vi "PVS Calibration.vi"(8 "Error In":errorcluster, 10 "Config PVS.AVOUT":dbl, 11 "TSM Context":T1) -> (0 "Error Out":errorcluster)   [LabVIEW 2019]
doc: "This VI use for Precision Voltage Source Calibration"
uses:
  <vilib>/NI_TestStand_SemiconductorModule/NI_TestStand_Semiconductor_Module.lvlibp/PinMap/General/SemiconductorModuleContext.ctl
  Common/Instrument Control/DMM/Pin Map/TSM DMM.ctl
  <vilib>/NI_TestStand_SemiconductorModule/NI_TestStand_Semiconductor_Module.lvlibp/PinMap/PinQueryContext/MultiplePinMultipleSessionQueryContext/MultiplePinMultipleSessionQueryContext.lvclass
  Common/Instrument Control/Relay/Pin Map/TSM Relay.ctl
  Common/Instrument Control/DCPower/TSM/TSM SSC DCPower.ctl
  Common/Instrument Control/DCPower/SSC DCPower/SSC DCPower.ctl
  Common/Instrument Control/Shared SubVIs/TSM Pin Abstraction/TSM Pin Information.ctl
  Common/Instrument Control/Shared SubVIs/TSM Pin Abstraction/TSM Pin Type Identifier.ctl
  Common/Instrument Control/Shared SubVIs/TSM Pin Abstraction/TSM Expanded Pin Information.ctl
  Common/Utility/typedefs/set_refdac_param.ctl
  <instrlib>/niDMM/nidmm.llb/niDMM Function.ctl
  <instrlib>/niDMM/nidmm.llb/niDMM Resolution in Digits.ctl
  <vilib>/NI_TestStand_SemiconductorModule/NI_TestStand_Semiconductor_Module.lvlibp/1abvi3w/instr.lib/niSwitch/niswitch.llb/niSwitch Relay Action.ctl
  <vilib>/NI_TestStand_SemiconductorModule/NI_TestStand_Semiconductor_Module.lvlibp
panel:
  out "ADC Voltage Out":dbl[](array[numeric])
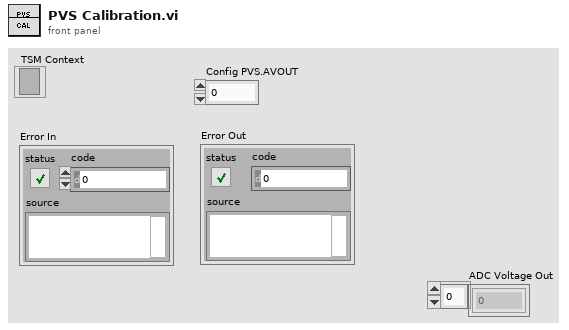
[diagram p1: front panel]
types:
  T1 = typedef "NI_TestStand_Semiconductor_Module.lvlibp/SemiconductorModuleContext.ctl" = refnum<k7>
  T2 = typedef "set_refdac_param.ctl" = cluster{"Read/Write":u16, "VREFP":dbl, "Select Register":enum16{"No Operation", "DAC Register", "Control Register", "Clearcode Register", "Software Control Register"}, "AVOUT ":dbl, "VREFN":dbl}
  T3 = typedef "TSM DMM.ctl" = cluster{"Pin Query Context":refnum<class "MultiplePinMultipleSessionQueryContext.lvclass">, "Sessions":refnum<k15>[]}
  T4 = typedef "TSM Relay.ctl" = cluster{"TSM Context":T1, "Relays":tag[]}
  T5 = typedef "TSM SSC DCPower.ctl" = cluster{"Pin Query Context":refnum<class "MultiplePinMultipleSessionQueryContext.lvclass">, "SSC":T6[], "Site Numbers":i32[], "Pins":T7[], "Pins Expanded":T9[]}
  T6 = typedef "SSC DCPower.ctl" = cluster{"Session":refnum<k15>, "Chan":string, "Channel List":string}
  T7 = typedef "TSM Pin Information.ctl" = cluster{"Pin":tag, "Type":T8, "Count":i32}
  T8 = typedef "TSM Pin Type Identifier.ctl" = enum8{"DUT Pin", "System Pin", "Pin Group", "Not Determined"}
  T9 = typedef "TSM Expanded Pin Information.ctl" = cluster{"Pin":tag, "Type":T8, "Index":i32}
  T10 = cluster{"DMM_Meas":T3, "PVS Cal Relay":T4, "SMU4139_V_OFFSET":T5}
  T11 = typedef "niDMM Function.ctl" = enum16{"DC Volts", "AC Volts", "DC Current", "AC Current", "2-wire Resistance", "4-wire Resistance", "Diode", "Frequency", "Period", "AC Volts DC Coupled", "Capacitance", "Inductance", "Temperature"}
  T12 = enum16{"N/A", "100mV", "1V", "10V", "100V", "1000V"}
  T13 = typedef "niDMM Resolution in Digits.ctl" = dbl
  T14 = typedef "NI_TestStand_Semiconductor_Module.lvlibp/niSwitch Relay Action.ctl" = i32
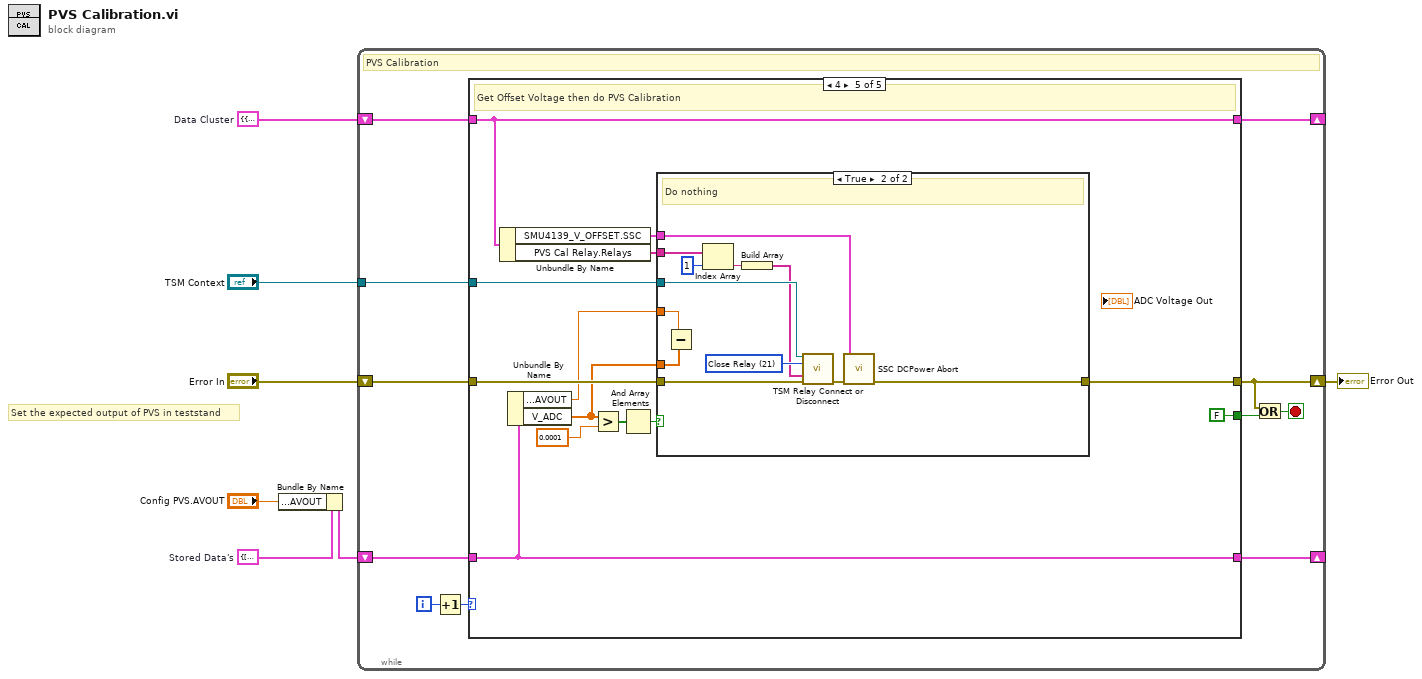
[diagram p0: block diagram]
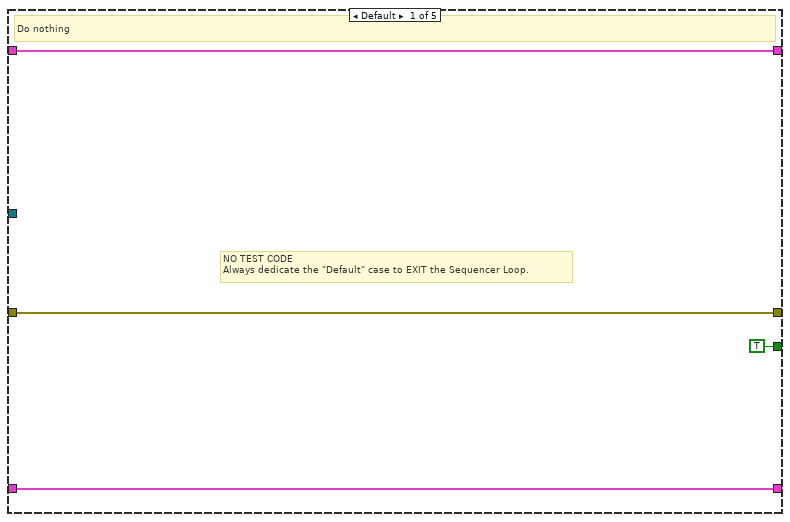
[diagram p2: hidden frame]
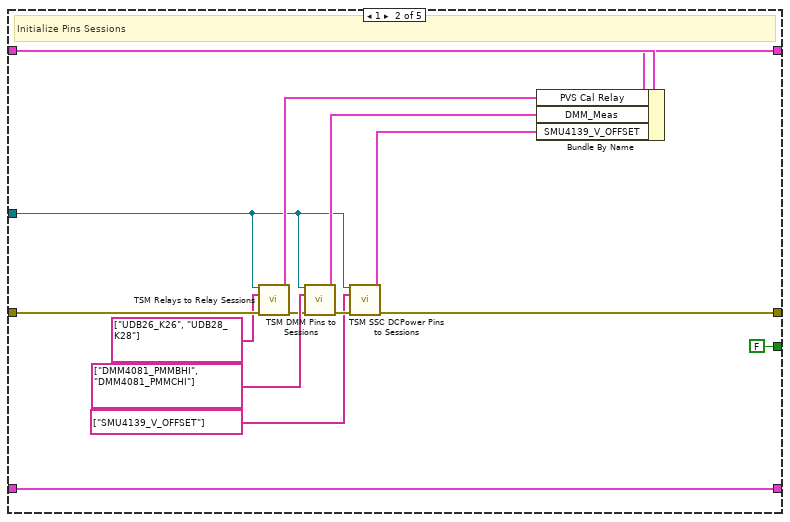
[diagram p3: hidden frame]
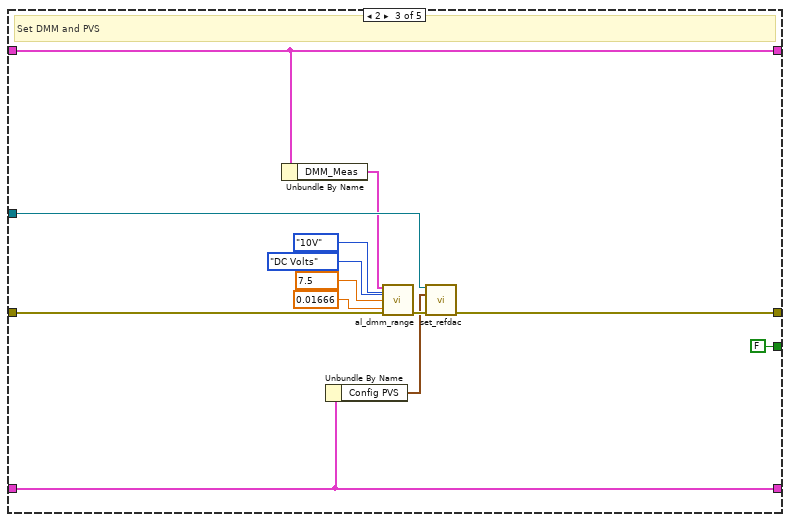
[diagram p4: hidden frame]
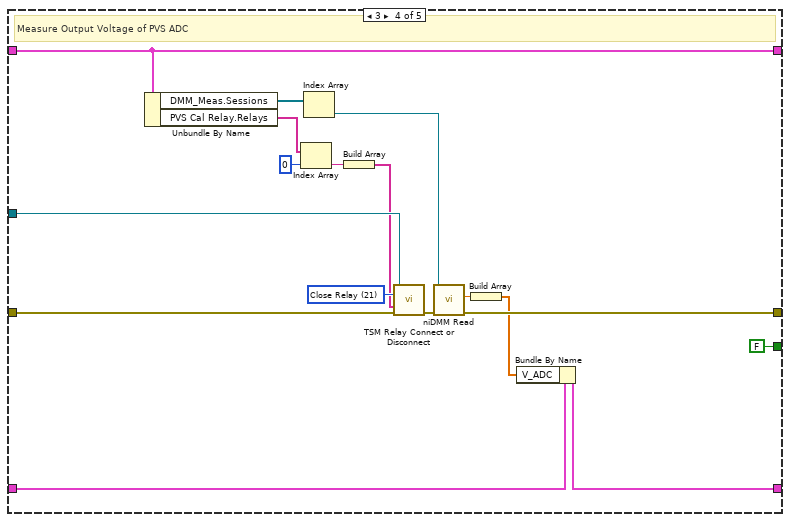
[diagram p5: hidden frame]
diagram:
  w3 = cluster{"V_ADC":dbl[], "Config PVS":T2} {"V_ADC"=[], "Config PVS"={"Read/Write"=0, "VREFP"=10.0, "Select Register"=enum."DAC Register", "AVOUT "=5.0, "VREFN"=-10.0}}  # Stored Data's
  w4 = T10 {"DMM_Meas"={"Pin Query Context"=refnum, "Sessions"=[]}, "PVS Cal Relay"={"TSM Context"=refnum, "Relays"=[]}, "SMU4139_V_OFFSET"={"Pin Query Context"=refnum, "SSC"=[], "Site Numbers"=[], "Pins"=[], "Pins Expanded"=[]}}  # Data Cluster
  # "Set the expected output of PVS in teststand"
  n1 = Bundle By Name(cluster=w3, "Config PVS.AVOUT"="Config PVS.AVOUT") -> (w2:cluster{"V_ADC":dbl[], "Config PVS":T2})
  n2 = while {
    tunnel: "TSM Context" -> [w15]
    shift-right: [w10] -> w5
    shift-left: "Error In" -> [w16]
    shift-right: [w13] -> _
    shift-left: w4 -> [w14]
    shift-right: [w11] -> _
    shift-left: w2 -> [w12]
    i -> [w18]
    stop <- w9 stop-if-true
    # "PVS Calibration"
    n3 = Increment(x=w18) -> (x+1=w17:i32)
    n4 = case shown="4" w17 {
      tunnel: w16 -> [w21 w33 w48 w65 w75]
      tunnel: w15 -> [_ w26 w49 w64 w68]
      tunnel: [w21 w23 w50 w62 w74] -> w10
      tunnel: w14 -> [w22 w36 w46 w67 w71]
      tunnel: [w22 w34 w46 w67 w71] -> w13
      tunnel: w12 -> [w20 w29 w39 w61 w79]
      tunnel: [w20 w29 w39 w60 w79] -> w11
      tunnel: [TRUE FALSE FALSE FALSE FALSE] -> w8
      frame Default {
        # "NO TEST CODE\nAlways dedicate the \"Default\" case to EXIT the Sequencer Loop."
        # "Do nothing"
      }
      frame 1 {
        # "Initialize Pins Sessions"
        n5 = call "TSM Relays to Relay Sessions.vi"("TSM Context"=w26, "Relays"=tag[] ["UDB26_K26", "UDB28_K28"], "error in (no error)"=w33) -> ("TSM Relay Out"=w30:T4, "error out"=w32:errorcluster)  [unwired: 11 in]
        n6 = call "TSM DMM Pins to Sessions.vi"("TSM Context"=w26, "Pins"=tag[] ["DMM4081_PMMBHI", "DMM4081_PMMCHI"], "error in"=w32) -> ("DMM TSM Out"=w35:T3, "error out"=w27:errorcluster)  [unwired: 11 in]
        n7 = call "TSM SSC DCPower Pins to Sessions.vi"("TSM context"=w26, "Pins"=tag[] ["SMU4139_V_OFFSET"], "error in"=w27) -> ("DCPower TSM Out"=w24:T5, "error out"=w23:errorcluster)  [unwired: 11 in]
        n8 = Bundle By Name(cluster=w36, "PVS Cal Relay"=w30, "DMM_Meas"=w35, "SMU4139_V_OFFSET"=w24) -> (w34:T10)
      }
      frame 2 {
        w41 = T13 7.5 items=["3 1/2"=3.5, "4 1/2"=4.5, "5 1/2"=5.5, "6 1/2"=6.5, "7 1/2"=7.5] ("Resolution in Digits")
        # "Set DMM and PVS"
        n9 = Unbundle By Name(w46) -> ("DMM_Meas"=w45:T3)
        n10 = Unbundle By Name(w39) -> ("Config PVS"=w38:T2)
        n11 = call "al_dmm_range.vi"("DMM TSM In"=w45, "DC Voltage Range"=T12."10V", "Function"=niDMM_Function."DC Volts", "Resolution in Digits"=w41, "error in"=w48, "Aperture Time (s)"=0.01666) -> ("error out"=w47:errorcluster)  [unwired: 9 in]
        n12 = call "set_refdac.vi"("TSM context"=w49, "Config PVS"=w38, "Error In"=w47) -> ("Error Out"=w50:errorcluster)  [unwired: 11 in, 1 out]
      }
      frame 3 {
        w58 = T14 21 items=["Open Relay"=20, "Close Relay"=21] ("Relay Action")
        # "Measure Output Voltage of PVS ADC"
        n13 = Unbundle By Name(w67) -> ("DMM_Meas.Sessions"=w66:refnum<k15>[], "PVS Cal Relay.Relays"=w63:tag[])
        n14 = Index Array(array=w63, index=0) -> (element=w56:tag)
        n15 = Index Array(array=w66) -> (element=w54:refnum<k15>)  [unwired: 1 in]
        n16 = Build Array(w56) -> (w55:tag[])
        n17 = call "TSM Relay Connect or Disconnect.vi"("TSM context"=w64, "Relay Action"=w58, "Relays"=w55, "error in"=w65) -> ("error out"=w57:errorcluster)  [unwired: 10 in, 1 out]
        n18 = call <instrlib>:"niDMM Read.vi"("error in (no error)"=w57, "instrument handle"=w54) -> ("error out"=w62:errorcluster, "Measurement"=w53:dbl)  [unwired: 7 in, 1 out]
        n19 = Build Array(w53) -> (w52:dbl[])
        n20 = Bundle By Name(cluster=w61, "V_ADC"=w52) -> (w60:cluster{"V_ADC":dbl[], "Config PVS":T2})
      }
      frame 4 {
        # "Get Offset Voltage then do PVS Calibration"
        n21 = Unbundle By Name(w71) -> ("SMU4139_V_OFFSET.SSC"=w70:T6[], "PVS Cal Relay.Relays"=w69:tag[])
        n22 = Unbundle By Name(w79) -> ("Config PVS.AVOUT"=w73:dbl, "V_ADC"=w72:dbl[])
        n23 = Greater?(x=w72, y=0.0001) -> (0:w77:bool[])
        n24 = And Array Elements(Boolean array=w77) -> (logical AND=w76:bool)
        n25 = case shown="True" w76 {
          tunnel: w75 -> [w81 w85]
          tunnel: [w81 w91] -> w74
          tunnel: w73 -> [_ w92]
          tunnel: w72 -> [_ w93]
          tunnel: w70 -> [_ w90]
          tunnel: w69 -> [_ w89]
          tunnel: w68 -> [_ w83]
          frame False {
            # "Do PVS Calibration"
          }
          frame True {
            w87 = T14 21 items=["Open Relay"=20, "Close Relay"=21] ("Relay Action")
            # "Do nothing"
            n26 = Subtract(x=w93, y=w92) -> ()  [unwired: 1 out]
            n27 = Index Array(array=w89, index=1) -> (element=w86:tag)
            n28 = Build Array(w86) -> (w82:tag[])
            n29 = call "TSM Relay Connect or Disconnect.vi"("TSM context"=w83, "Relay Action"=w87, "Relays"=w82, "error in"=w85) -> ("error out"=w84:errorcluster)  [unwired: 10 in, 1 out]
            n30 = call "SSC DCPower Abort.vi"("DCPower SSC in"=w90, "error in"=w84) -> ("error out"=w91:errorcluster)  [unwired: 12 in, 1 out]
          }
        }
      }
    }
    n31 = Or(x=w10, y=w8) -> (x .or. y?=w9:bool)
  }
  "Error Out" <- w5
